vi "Menu-Start Log.vi"(8 "error in (no error)":errorcluster, 11 "Menu in":refnum<k9>) -> ()   [LabVIEW 2016, in "CML UI.lvlib"]
uses:
  CML UI.lvlib
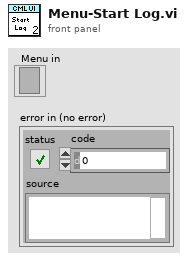
[diagram p1: front panel]
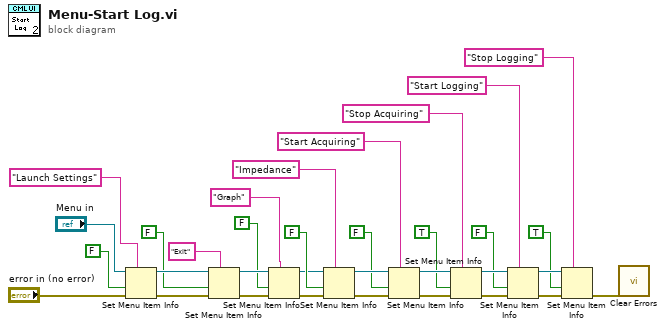
[diagram p0: block diagram]
diagram:
  n1 = Set Menu Item Info(7:"Launch Settings" ("item tag"), 8:"error in (no error)", 9:FALSE ("enabled"), 11:"Menu in") -> (0:w16:errorcluster, 3:w17:refnum<k9>)  [unwired: 3 in]
  n2 = Set Menu Item Info(7:"Exit" ("item tag"), 8:w16, 9:FALSE ("enabled"), 11:w17) -> (0:w29:errorcluster, 3:w28:refnum<k9>)  [unwired: 3 in]
  n3 = Set Menu Item Info(7:"Graph" ("item tag"), 8:w29, 9:FALSE ("enabled"), 11:w28) -> (0:w27:errorcluster, 3:w22:refnum<k9>)  [unwired: 3 in]
  n4 = Set Menu Item Info(7:"Impedance" ("item tag"), 8:w27, 9:FALSE ("enabled"), 11:w22) -> (0:w31:errorcluster, 3:w30:refnum<k9>)  [unwired: 3 in]
  n5 = Set Menu Item Info(7:"Start Acquiring" ("item tag"), 8:w31, 9:FALSE ("enabled"), 11:w30) -> (0:w20:errorcluster, 3:w21:refnum<k9>)  [unwired: 3 in]
  n6 = Set Menu Item Info(7:"Stop Acquiring" ("item tag"), 8:w20, 9:TRUE ("enabled"), 11:w21) -> (0:w4:errorcluster, 3:w12:refnum<k9>)  [unwired: 3 in]
  n7 = Set Menu Item Info(7:"Start Logging" ("item tag"), 8:w4, 9:FALSE ("enabled"), 11:w12) -> (0:w5:errorcluster, 3:w13:refnum<k9>)  [unwired: 3 in]
  n8 = Set Menu Item Info(7:"Stop Logging" ("item tag"), 8:w5, 9:TRUE ("enabled"), 11:w13) -> (0:w1:errorcluster)  [unwired: 3 in, 1 out]
  n9 = call <vilib>:"Clear Errors.vi"("error in (no error)"=w1) -> ()  [unwired: 5 in, 2 out]
